vi "Joystick Controls to Commands.vi"(11 "Robot Controls":T2) -> (3 "Robot Commands":T1)   [LabVIEW 2014]
uses:
  Subsystem VIs/Robot Control Outputs.ctl
  Subsystem VIs/Robot Commands.ctl
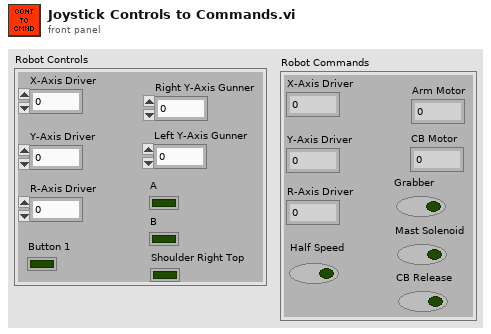
[diagram p1: front panel]
types:
  T1 = typedef "Robot Commands.ctl" = cluster{"X-Axis Driver":dbl, "Y-Axis Driver":dbl, "R-Axis Driver":dbl, "Arm Motor":dbl, "CB Motor":dbl, "Grabber":bool, "Mast Solenoid":bool, "CB Release":bool, "Half Speed":bool}
  T2 = typedef "Robot Control Outputs.ctl" = cluster{"X-Axis Driver":dbl, "Y-Axis Driver":dbl, "R-Axis Driver":dbl, "Button 1":bool, "Right Y-Axis Gunner":dbl, "Left Y-Axis Gunner":dbl, "A":bool, "B":bool, "Shoulder Right Top ":bool}
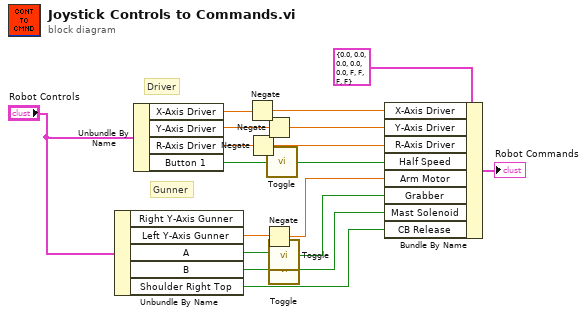
[diagram p0: block diagram]
diagram:
  # "Gunner"
  # "Driver"
  n1 = Unbundle By Name("Robot Controls") -> ("Left Y-Axis Gunner"=w13:dbl, "A"=w12:bool, "B"=w11:bool, "Shoulder Right Top"=w3:bool)  [unwired: 1 out]
  n2 = Unbundle By Name("Robot Controls") -> ("X-Axis Driver"=w17:dbl, "Y-Axis Driver"=w16:dbl, "R-Axis Driver"=w15:dbl, "Button 1"=w14:bool)
  n3 = Negate(x=w17) -> (-x=w10:dbl)
  n4 = Negate(x=w15) -> (-x=w8:dbl)
  n5 = Negate(x=w16) -> (-x=w9:dbl)
  n6 = Negate(x=w13) -> (-x=w6:dbl)
  n7 = call "Toggle.vi"("Input"=w14) -> ("Output"=w7:bool)
  n8 = call "Toggle.vi"("Input"=w12) -> ("Output"=w5:bool)
  n9 = call "Toggle.vi"("Input"=w11) -> ("Output"=w4:bool)
  n10 = Bundle By Name(cluster=T1 {"X-Axis Driver"=0.0, "Y-Axis Driver"=0.0, "R-Axis Driver"=0.0, "Arm Motor"=0.0, "CB Motor"=0.0, "Grabber"=FALSE, "Mast Solenoid"=FALSE, "CB Release"=FALSE, "Half Speed"=FALSE} ("Robot Controls"), "X-Axis Driver"=w10, "Y-Axis Driver"=w9, "R-Axis Driver"=w8, "Half Speed"=w7, "Arm Motor"=w6, "Grabber"=w5, "Mast Solenoid"=w4, "CB Release"=w3) -> (→"Robot Commands":T1)
